vi "Controller Status Table.vi"() -> ()   [LabVIEW 2011, in "Controller Global Variables.lvlib"]
uses:
  Controller Global Variables.lvlib
panel:
  in  "Controller Status Table":i32[](array[numeric])
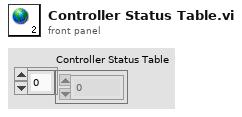
[diagram p1: front panel]
diagram:
